vi "populate_index.vi"(8 "error in (no error)":errorcluster, 10 "variable_info_in":T1) -> (0 "error out":errorcluster, 2 "variable_info_out":T1)   [LabVIEW 2015, in "Scan Engine runtime.lvclass"]
uses:
  Scan Engine runtime.lvclass
  Custom Ctrls/Index Map.ctl
  <vilib>/NI/Tag Bus/tag/Data Type.ctl
  <resource>/objmgr/ni.var.rc
  <vilib>/NI/Tag Bus/tag/tag descriptor.lvclass
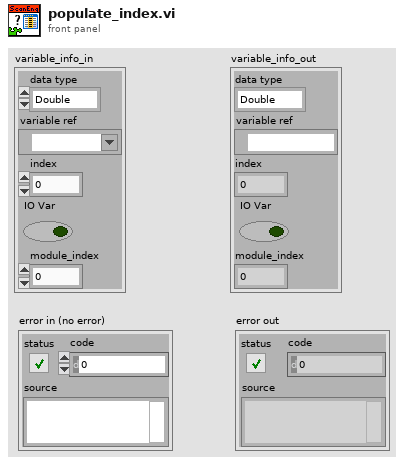
[diagram p1: front panel]
types:
  T1 = typedef "Scan Engine runtime.lvclass/Index Map.ctl" = cluster{"data type":T2, "variable ref":refnum<k21>, "index":i32, "IO Var":bool, "module_index":i32}
  T2 = typedef "tag bus.lvlib/tag descriptor.lvclass/Data Type.ctl" = enum16{"Double", "Single", "I64", "I32", "I16", "I8", "U64", "U32", "U16", "U8", "Boolean", "String", "Array of Double", "Array of Single", "Array of I64", "Array of I32", "Array of I16", "Array of I8", "Array of U64", "Array of U32", "Array of U16", "Array of U8", "Array of Boolean", "Array of String"}
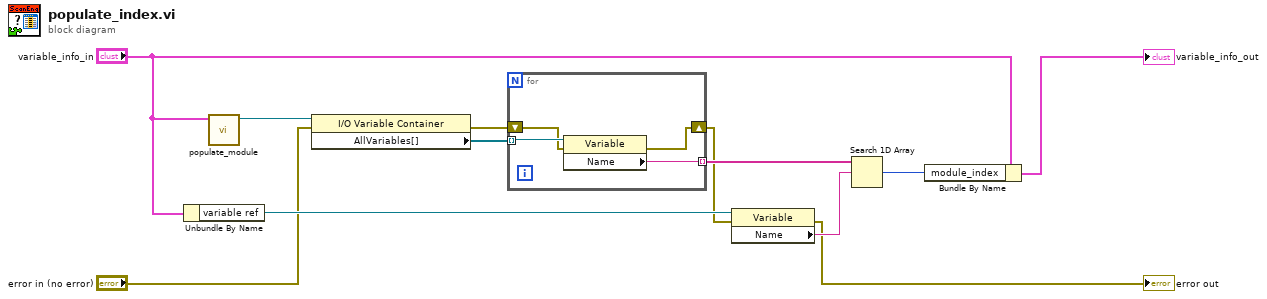
[diagram p0: block diagram]
diagram:
  n1 = Unbundle By Name("variable_info_in") -> ("variable ref"=w11:refnum<k21>)
  n2 = call "populate_module.vi"("variable_info_in"="variable_info_in") -> ("Module"=w5:refnum<k21>)  [unwired: 10 in]
  n3 = property class="I/O Variable Container"(reference=w5, error in="error in (no error)") -> (error out=w3:errorcluster, "AllVariables[]"=w9:refnum<k21>[])  [unwired: 1 out]
  n4 = for {
    tunnel: w9 -> [w16] mode=indexing
    tunnel: [w15] -> w10 mode=indexing
    shift-right: [w13] -> w2
    shift-left: w3 -> [w14]
    n5 = property class="Variable"(reference=w16, error in=w14) -> (error out=w13:errorcluster, "Name"=w15:string)  [unwired: 1 out]
  }
  n6 = property class="Variable"(reference=w11, error in=w2) -> (error out=→"error out":errorcluster, "Name"=w12:string)  [unwired: 1 out]
  n7 = Search 1D Array(1D array=w10, element=w12) -> (index of element=w8:i32)  [unwired: 1 in]
  n8 = Bundle By Name(cluster="variable_info_in", "module_index"=w8) -> (→"variable_info_out":T1)
